vi "aquireAPRS.vi"() -> ()   [LabVIEW 2012]
panel:
  out "Single String":string
  in  "attempt to filter":bool
  in  "Password":string
  in  "callsign for filter":string
  in  "stop":bool
  out "Raw Data":string
  in  "Login":string
  in  "port":dbl
  in  "server":string
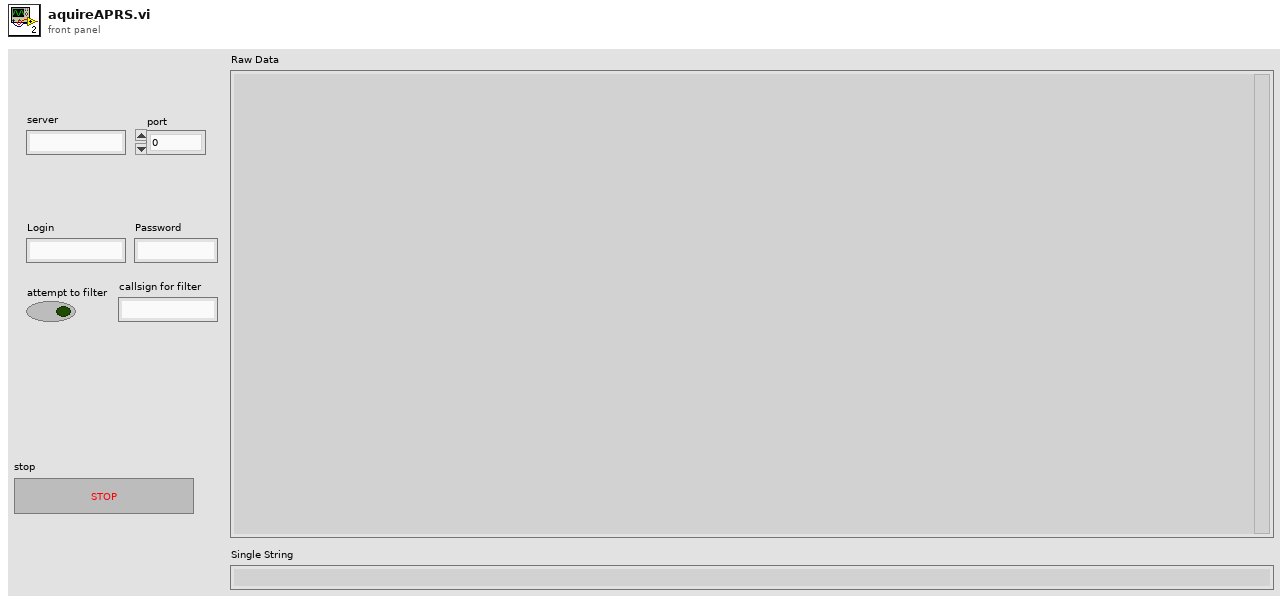
[diagram p1: front panel]
types:
  T1 = enum16{"Standard", "Buffered", "CRLF", "Immediate"}
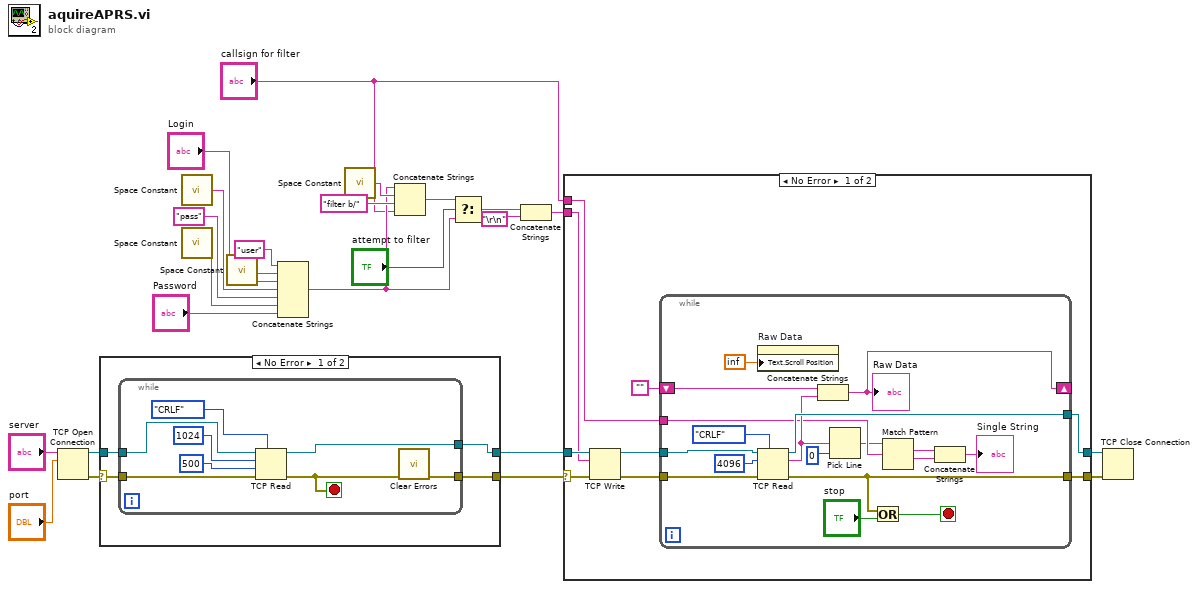
[diagram p0: block diagram]
diagram:
  n1 = TCP Open Connection(address="server", remote port or service name="port") -> (connection ID=w22:refnum<k5>, error out=w23:errorcluster)  [unwired: 3 in]
  n2 = case shown="No Error" w23 {
    selector: w23 -> [w27 w38]
    tunnel: w22 -> [w28 w37]
    tunnel: [w25 w38] -> w7
    tunnel: [w26 w37] -> w8
    frame No Error {
      n3 = while {
        tunnel: w28 -> [w36]
        tunnel: [w35] -> w26
        tunnel: w27 -> [w34]
        tunnel: [w30] -> w25
        stop <- w29 stop-if-true
        n4 = TCP Read(connection ID=w36, bytes to read=1024, error in (no error)=w34, 7:T1."CRLF" ("mode (standard)"), 9:500 ("timeout ms (25000)")) -> (connection ID out=w35:refnum<k5>, error out=w29:errorcluster)  [unwired: 1 out]
        n5 = call <vilib>:"Clear Errors.vi"("error in (no error)"=w29) -> ("error out"=w30:errorcluster)  [unwired: 6 in]
      }
    }
    frame Error {
    }
  }
  n6 = call <vilib>:"Space Constant.vi"() -> ("String"=w14:string)
  n7 = call <vilib>:"Space Constant.vi"() -> ("String"=w13:string)
  n8 = call <vilib>:"Space Constant.vi"() -> ("String"=w16:string)
  n9 = Concatenate Strings("user", w16, "Login", w14, "pass" ("string"), w13, "Password") -> (w9:string)
  n10 = call <vilib>:"Space Constant.vi"() -> ("String"=w17:string)
  n11 = Concatenate Strings(w9, w17, "filter b/" ("string"), "callsign for filter") -> (w10:string)
  n12 = Select(t=w10, s="attempt to filter", f=w9) -> (s? t:f=w3:string)
  n13 = Concatenate Strings(w3, "\r\n") -> (w4:string)
  n14 = case shown="No Error" w7 {
    selector: w7 -> [w43 w66]
    tunnel: w8 -> [w44 w67]
    tunnel: [w42 w67] -> w6
    tunnel: [w41 w66] -> w5
    tunnel: w4 -> [w40 _]
    tunnel: "callsign for filter" -> [w39 _]
    frame No Error {
      n15 = TCP Write(connection ID=w44, data in=w40, error in (no error)=w43) -> (connection ID out=w45:refnum<k5>, error out=w46:errorcluster)  [unwired: 1 in, 1 out]
      n16 = while {
        tunnel: w45 -> [w65]
        tunnel: w46 -> [w64]
        tunnel: [w59] -> w41
        tunnel: [w63] -> w42
        shift-right: [w56] -> _
        shift-left: "" -> [w61]
        tunnel: w39 -> [w52]
        stop <- w58 stop-if-true
        n17 = property on="Raw Data" class="Str"("Text.Scroll Position"=inf) -> ()  [unwired: 2 in, 2 out]
        n18 = TCP Read(connection ID=w65, bytes to read=4096, error in (no error)=w64, 7:T1."CRLF" ("mode (standard)")) -> (connection ID out=w63:refnum<k5>, data out=w54:string, error out=w59:errorcluster)  [unwired: 1 in]
        n19 = Concatenate Strings(w61, w54) -> (w56:string)
        "Raw Data" <- w56
        n20 = Pick Line(multi-line string=w54, line index=0) -> (output string=w51:string)  [unwired: 1 in]
        n21 = Or(x=w59, y="stop") -> (x .or. y?=w58:bool)
        n22 = Match Pattern(string=w51, regular expression=w52) -> (match substring=w50:string, after substring=w49:string)  [unwired: 1 in, 2 out]
        n23 = Concatenate Strings(w50, w49) -> (→"Single String":string)
      }
    }
    frame Error {
    }
  }
  n24 = TCP Close Connection(connection ID=w6, error in (no error)=w5) -> ()  [unwired: 1 in, 2 out]
